vi "setResetFF.vi"(8 "Set":bool, 10 "Reset":bool) -> (2 "Result":bool)   [LabVIEW 2010, in "KevLib01.lvlib"]
uses:
  KevLib01.lvlib
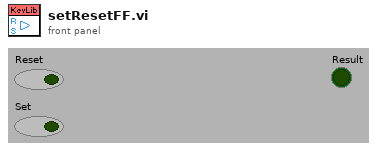
[diagram p1: front panel]
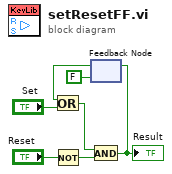
[diagram p0: block diagram]
diagram:
  n1 = Not(x="Reset") -> (.not. x?=w6:bool)
  n2 = feedback #1(FALSE) -> (w2:bool)
  n3 = Or(x=w2, y="Set") -> (x .or. y?=w7:bool)
  n4 = And(x=w7, y=w6) -> (x .and. y?=w3:bool)
  "Result" <- w3
  n5 = feedback-in #1(w3) -> ()
